vi "Expt_5-sqroot.vi"() -> ()   [LabVIEW 2020]
panel:
  out "Result":dbl
  in  "b":dbl
  in  "a":dbl
  in  "Mode":dbl
  out "current time":timestamp
  out "sqrt(x)":dbl
  in  "x":dbl
  # "1)"
  # "2)"
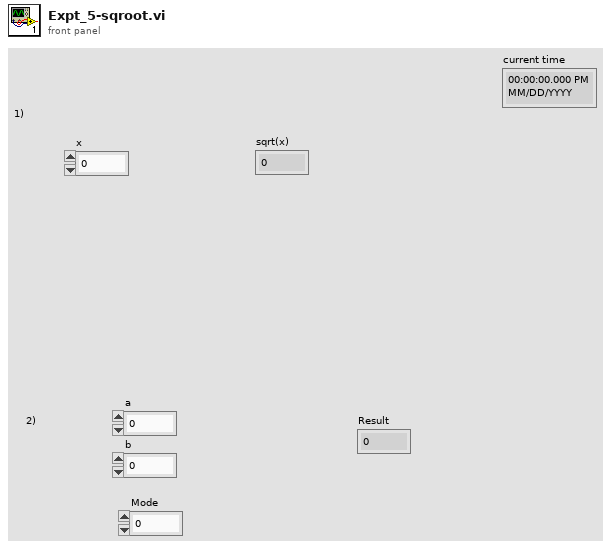
[diagram p1: front panel]
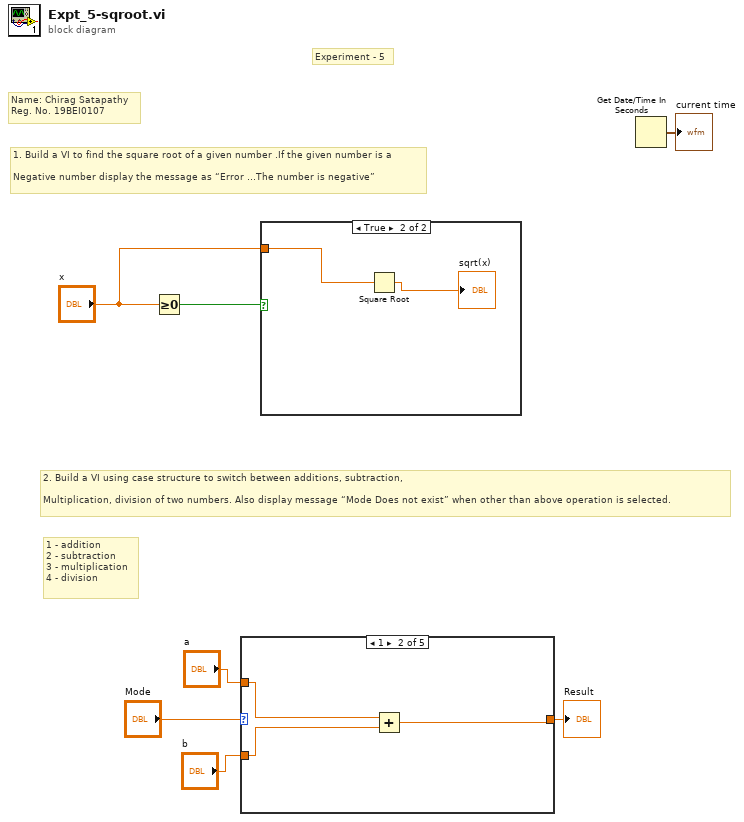
[diagram p0: block diagram]
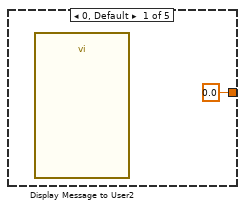
[diagram p2: hidden frame]
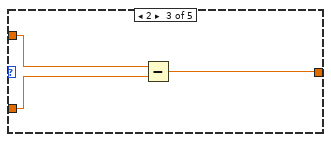
[diagram p3: hidden frame]
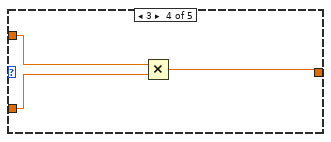
[diagram p4: hidden frame]
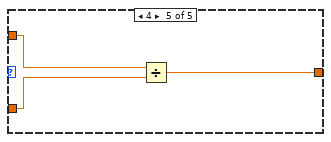
[diagram p5: hidden frame]
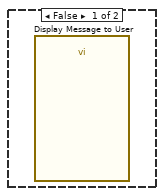
[diagram p6: hidden frame]
diagram:
  # "1 - addition\n2 - subtraction\n3 - multiplication\n4 - division"
  # "2. Build a VI using case structure to switch between additions, subtraction,\n\nMultiplication, division of two numbers. Also display message “Mode Does not exist” when other than above operation is selected."
  # "1. Build a VI to find the square root of a given number .If the given number is a\n\nNegative number display the message as “Error …The number is negative”"
  # "Name: Chirag Satapathy\nReg. No. 19BEI0107"
  # "Experiment - 5"
  n1 = Greater Or Equal To 0?(x="x") -> (x >= 0?=w7:bool)
  n2 = case shown="1" "Mode" {
    tunnel: "a" -> [_ w11 w14 w17 w20]
    tunnel: "b" -> [_ w10 w13 w16 w19]
    tunnel: [0.0 w9 w12 w15 w18] -> w1
    frame 0, Default {
      n3 = call "Display Message to User2"() -> ()  [unwired: 10 in, 2 out]
    }
    frame 1 {
      n4 = Add(x=w11, y=w10) -> (x+y=w9:dbl)
    }
    frame 2 {
      n5 = Subtract(x=w14, y=w13) -> (x-y=w12:dbl)
    }
    frame 3 {
      n6 = Multiply(x=w17, y=w16) -> (x*y=w15:dbl)
    }
    frame 4 {
      n7 = Divide(x=w20, y=w19) -> (x/y=w18:dbl)
    }
  }
  "Result" <- w1
  n8 = case shown="True" w7 {
    tunnel: "x" -> [_ w22]
    frame False {
      n9 = call "Display Message to User"() -> ()  [unwired: 10 in, 2 out]
    }
    frame True {
      n10 = Square Root(x=w22) -> (sqrt(x)=→"sqrt(x)":dbl)
    }
  }
  n11 = Get Date/Time In Seconds() -> (seconds since 1Jan1904=→"current time":timestamp)
